vi "Wait Client Loops Stopped.vi"(8 "error in (no error)":errorcluster, 11 "TCPMessaging in":refnum<class "TCPMessaging.lvclass">) -> (0 "error out":errorcluster, 3 "TCPMessaging out":refnum<class "TCPMessaging.lvclass">)   [LabVIEW 2020, in "Vecto.lvlib" / "TCPMessaging.lvclass"]
uses:
  TCPMessaging.lvclass
  TCPMessaging.lvclass/TCPMessaging.ctl
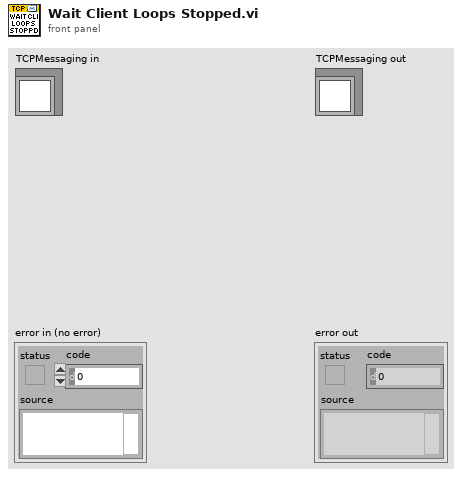
[diagram p1: front panel]
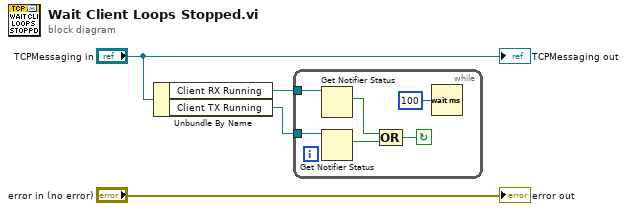
[diagram p0: block diagram]
diagram:
  n1 = Unbundle By Name("TCPMessaging in") -> ("Client RX Running"=w3:refnum<notifier>, "Client TX Running"=w2:refnum<notifier>)
  n2 = while {
    tunnel: w3 -> [w9]
    tunnel: w2 -> [w10]
    stop <- w8 continue-if-true
    n3 = Get Notifier Status(notifier=w9) -> (current notification=w6:bool)  [unwired: 1 in, 4 out]
    n4 = Get Notifier Status(notifier=w10) -> (current notification=w5:bool)  [unwired: 1 in, 4 out]
    n5 = Compound Arithmetic op=OR(w6, w5) -> (w8:bool)
    n6 = Wait (ms)(milliseconds to wait=u32 100) -> ()  [unwired: 1 out]
  }
  "error out" <- "error in (no error)"
  "TCPMessaging out" <- "TCPMessaging in"
